vi "Stop ILC.vi"(8 "error in (no error)":errorcluster, 11 "Model in":refnum<class "Model.lvclass">) -> (0 "error out":errorcluster, 3 "Model out":refnum<class "Model.lvclass">)   [LabVIEW 2016, in "Model.lvclass"]
uses:
  Model.lvclass
  Model.lvclass/Model.ctl
  Modbus/DesktopModbus/DesktopModbus.lvclass
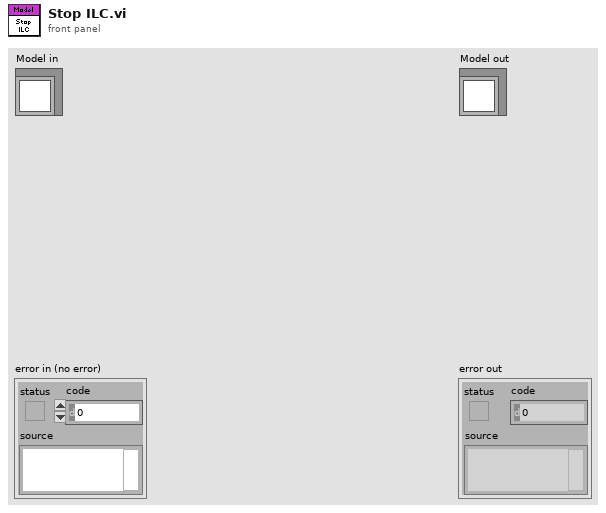
[diagram p1: front panel]
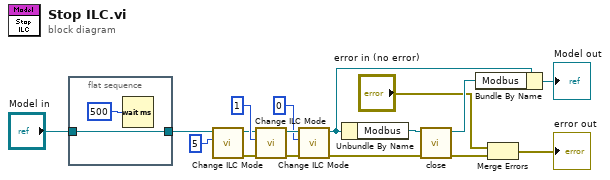
[diagram p0: block diagram]
diagram:
  n1 = flat-sequence {
    tunnel: "Model in" -> [w19]
    tunnel: [w19] -> w1
    frame #0 {
      n2 = Wait (ms)(milliseconds to wait=u32 500) -> ()  [unwired: 1 out]
    }
  }
  n3 = call "Change ILC Mode.vi"("Mode"=u16 5, "Model in"=w1) -> ("error out"=w17:errorcluster, "Model out"=w15:refnum<class "Model.lvclass">)  [unwired: 8 in]
  n4 = call "Change ILC Mode.vi"("error in (no error)"=w17, "Mode"=u16 1, "Model in"=w15) -> ("error out"=w6:errorcluster, "Model out"=w7:refnum<class "Model.lvclass">)  [unwired: 7 in]
  n5 = call "Change ILC Mode.vi"("error in (no error)"=w6, "Mode"=u16 0, "Model in"=w7) -> ("error out"=w3:errorcluster, "Model out"=w4:refnum<class "Model.lvclass">)  [unwired: 7 in]
  n6 = Unbundle By Name(w4) -> ("Modbus"=w11:refnum<class "DesktopModbus.lvclass">)
  n7 = call "close.vi"("error in (no error)"=w3, "DesktopModbus in"=w11) -> ("error out"=w13:errorcluster, "DesktopModbus out"=w12:refnum<class "DesktopModbus.lvclass">)  [unwired: 8 in]
  n8 = Bundle By Name(cluster=w4, "Modbus"=w12) -> (→"Model out":refnum<class "Model.lvclass">)
  n9 = Merge Errors("error in (no error)", w13) -> (→"error out":errorcluster)
